vi "UHR-Fleezers Control (host) - Lorentz v2.vi"() -> ()   [LabVIEW 2014] (continued)
          tunnel: "Inject Pump 2" -> [_ w2660]
          frame False {
          }
          frame True {
            n1765 = local read "Flow rate (uL/h)"() -> (w2654:dbl)
            n1766 = Number To Decimal String(number=w2654) -> (decimal integer string=w2656:string)  [unwired: 1 in]
            n1767 = Concatenate Strings("on, flow rate", w2656) -> (w2655:string)
            n1768 = Select(t=w2655, s=w2660, f="off") -> (s? t:f=w2664:string)
            n1769 = local read "Time (s)"() -> (w2658:dbl)
            n1770 = local read "log file ref"() -> (w2659:refnum<file>)
            n1771 = Concatenate Strings("pump 2 ", w2664) -> (w2662:string)
            n1772 = call "write to event log.vi"("log file ref"=w2659, "time"=w2658, "input string"=w2662) -> ()  [unwired: 8 in]
          }
        }
      }
      event "Sample Channel\nFlow": Value Change {
        n1773 = event-data() -> ()  [unwired: 7 out]
        n1774 = disable-structure shown="Disabled" {
          disable-tunnel: w2682 -> [w2689 _]
          frame Disabled {
            n1775 = Select(t="irun" ("string"), s="Sample Channel\nFlow", f="stop" ("string")) -> (s? t:f=w2684:string)
            n1776 = Concatenate Strings(w2684, "\r") -> (w2687:string)
            n1777 = VISA Write(VISA resource name=w2689, write buffer=w2687) -> ()  [unwired: 1 in, 3 out]
          }
          frame Enabled {
          }
        }
      }
      event "Start Flow": Value Change {
        n1778 = event-data() -> ()  [unwired: 7 out]
        n1779 = disable-structure shown="Disabled" {
          disable-tunnel: w2690 -> [w2691 _]
          frame Disabled {
            n1780 = local write "Sample Channel\nFlow"(TRUE ("Sample Channel\nFlow")) -> ()
            n1781 = local write "Start Flow"(FALSE ("Start Flow")) -> ()
            n1782 = Concatenate Strings("irun" ("string"), "\r") -> (w2695:string)
            n1783 = VISA Write(VISA resource name=w2691, write buffer=w2695) -> ()  [unwired: 1 in, 3 out]
          }
          frame Enabled {
          }
        }
      }
      event "Stop Flow": Value Change {
        n1784 = event-data() -> ()  [unwired: 7 out]
        n1785 = disable-structure shown="Disabled" {
          disable-tunnel: w2697 -> [w2699 _]
          frame Disabled {
            w2698 = FALSE ("Stop Flow")
            n1786 = local write "Stop Flow"(w2698) -> ()
            n1787 = local write "Sample Channel\nFlow"(w2698) -> ()
            n1788 = Concatenate Strings("stop" ("string"), "\r") -> (w2701:string)
            n1789 = VISA Write(VISA resource name=w2699, write buffer=w2701) -> ()  [unwired: 1 in, 3 out]
          }
          frame Enabled {
          }
        }
      }
      event "Flow rate (uL/h)": Value Change {
        n1790 = event-data() -> ()  [unwired: 7 out]
        n1791 = disable-structure shown="Disabled" {
          disable-tunnel: w2703 -> [w2705 _]
          frame Disabled {
            n1792 = Number To Decimal String(number="Flow rate (uL/h)") -> (decimal integer string=w2709:string)  [unwired: 1 in]
            n1793 = Concatenate Strings("irate  " ("string"), w2709, " u/h" ("string"), "\r") -> (w2708:string)
            n1794 = VISA Write(VISA resource name=w2705, write buffer=w2708) -> ()  [unwired: 1 in, 3 out]
          }
          frame Enabled {
          }
        }
      }
      event "Flush Sample": Value Change {
        n1795 = event-data() -> ()  [unwired: 7 out]
        n1796 = disable-structure shown="Disabled" {
          disable-tunnel: ["Flush Sample" _] -> w2712
          disable-tunnel: w2711 -> [w2718 _]
          frame Disabled {
            n1797 = flat-sequence {
              tunnel: w2718 -> [w2759]
              tunnel: [w2739] -> w2722
              tunnel: [w2735] -> w2721
              tunnel: ["Volume (uL)"] -> w2717
              tunnel: ["Flush rate (uL/m)"] -> w2716
              tunnel: w2722 -> [w2763]
              tunnel: [w2763] -> w2720
              tunnel: w2721 -> [w2762]
              tunnel: w2720 -> [w2768]
              frame #0 {
                # "set paramaters (rate, volume) for flush, clear volume"
                n1798 = Number To Decimal String(number="Flush rate (uL/m)") -> (decimal integer string=w2755:string)  [unwired: 1 in]
                n1799 = Concatenate Strings("irate  " ("string"), w2755, " u/m" ("string"), "\r") -> (w2757:string)
                n1800 = VISA Write(VISA resource name=w2759, write buffer=w2757) -> (VISA resource name out=w2753:refnum<visa-resource-name>)  [unwired: 1 in, 2 out]
                n1801 = Reciprocal(x="Flush rate (uL/m)") -> (1/x=w2738:dbl)
                n1802 = Number To Decimal String(number="Volume (uL)") -> (decimal integer string=w2744:string)  [unwired: 1 in]
                n1803 = Multiply(x="Volume (uL)", y=w2738) -> (x*y=w2737:dbl)
                n1804 = Concatenate Strings("tvolume  " ("string"), w2744, " u" ("string"), "\r") -> (w2742:string)
                n1805 = Multiply(x=w2737, y=60000.0) -> (x*y=w2735:dbl)
                n1806 = VISA Write(VISA resource name=w2753, write buffer=w2742) -> (VISA resource name out=w2741:refnum<visa-resource-name>)  [unwired: 1 in, 2 out]
                n1807 = Concatenate Strings("cvolume" ("string"), "\r") -> (w2740:string)
                n1808 = VISA Write(VISA resource name=w2741, write buffer=w2740) -> (VISA resource name out=w2751:refnum<visa-resource-name>)  [unwired: 1 in, 2 out]
                n1809 = Concatenate Strings("irun" ("string"), "\r") -> (w2749:string)
                n1810 = VISA Write(VISA resource name=w2751, write buffer=w2749) -> (VISA resource name out=w2739:refnum<visa-resource-name>)  [unwired: 1 in, 2 out]
              }
              frame #1 {
                # "Have to wait until\nflow is done to reset\nrate"
                n1811 = Add(x=w2762, y=100.0) -> (x+y=w2761:dbl)
                n1812 = Wait (ms)(milliseconds to wait=w2761) -> ()  [unwired: 1 out]
              }
              frame #2 {
                # "reset flow rate to usual flow rate"
                n1813 = local read "Flow rate (uL/h)"() -> (w2774:dbl)
                n1814 = Number To Decimal String(number=w2774) -> (decimal integer string=w2772:string)  [unwired: 1 in]
                n1815 = Concatenate Strings("irate  " ("string"), w2772, " u/h" ("string"), "\r") -> (w2770:string)
                n1816 = VISA Write(VISA resource name=w2768, write buffer=w2770) -> (VISA resource name out=w2764:refnum<visa-resource-name>)  [unwired: 1 in, 2 out]
                n1817 = Concatenate Strings("cvolume" ("string"), "\r") -> (w2765:string)
                n1818 = VISA Write(VISA resource name=w2764, write buffer=w2765) -> ()  [unwired: 1 in, 3 out]
              }
            }
            n1819 = local read "Save Event Log?"() -> (w2714:bool)
            n1820 = local read "Saving..."() -> (w2713:bool)
            n1821 = And(x=w2714, y=w2713) -> (x .and. y?=w2715:bool)
            n1822 = case shown="True" w2715 {
              tunnel: w2717 -> [_ w2724]
              tunnel: w2716 -> [_ w2723]
              frame False {
              }
              frame True {
                n1823 = Number To Decimal String(number=w2724) -> (decimal integer string=w2728:string)  [unwired: 1 in]
                n1824 = Number To Decimal String(number=w2723) -> (decimal integer string=w2730:string)  [unwired: 1 in]
                n1825 = local read "log file ref"() -> (w2725:refnum<file>)
                n1826 = local read "Time (s)"() -> (w2726:dbl)
                n1827 = Concatenate Strings("pump 2 flushing ", w2728, " uL at ", w2730, " ul/min") -> (w2732:string)
                n1828 = call "write to event log.vi"("log file ref"=w2725, "time"=w2726, "input string"=w2732) -> ()  [unwired: 8 in]
              }
            }
          }
          frame Enabled {
          }
        }
      }
      event "Flush Pump 3": Value Change {
        n1829 = event-data() -> ()  [unwired: 7 out]
        n1830 = disable-structure shown="Disabled" {
          disable-tunnel: ["Flush Pump 3" _] -> w2776
          disable-tunnel: w2775 -> [w2782 _]
          frame Disabled {
            n1831 = flat-sequence {
              tunnel: w2782 -> [w2797]
              tunnel: ["Flush rate (uL/m) P3"] -> w2778
              tunnel: ["Volume (uL) P3"] -> w2777
              frame #0 {
                # "set paramaters (rate, volume) for flush, clear volume"
                n1832 = Number To Decimal String(number="Flush rate (uL/m) P3") -> (decimal integer string=w2817:string)  [unwired: 1 in]
                n1833 = local write "Inject Pump 3"(TRUE ("Inject Pump 3")) -> ()
                n1834 = Concatenate Strings("irate  " ("string"), w2817, " u/m" ("string"), "\r") -> (w2819:string)
                n1835 = VISA Write(VISA resource name=w2797, write buffer=w2819) -> (VISA resource name out=w2815:refnum<visa-resource-name>)  [unwired: 1 in, 2 out]
                n1836 = Reciprocal(x="Flush rate (uL/m) P3") -> (1/x=w2801:dbl)
                n1837 = Number To Decimal String(number="Volume (uL) P3") -> (decimal integer string=w2806:string)  [unwired: 1 in]
                n1838 = Multiply(x="Volume (uL) P3", y=w2801) -> (x*y=w2800:dbl)
                n1839 = Concatenate Strings("tvolume  " ("string"), w2806, " u" ("string"), "\r") -> (w2804:string)
                n1840 = Multiply(x=w2800, y=60.0) -> (x*y=→"HP3 Flush Time (s)":dbl)
                n1841 = VISA Write(VISA resource name=w2815, write buffer=w2804) -> (VISA resource name out=w2803:refnum<visa-resource-name>)  [unwired: 1 in, 2 out]
                n1842 = Concatenate Strings("cvolume" ("string"), "\r") -> (w2802:string)
                n1843 = VISA Write(VISA resource name=w2803, write buffer=w2802) -> (VISA resource name out=w2813:refnum<visa-resource-name>)  [unwired: 1 in, 2 out]
                n1844 = Concatenate Strings("irun" ("string"), "\r") -> (w2811:string)
                n1845 = VISA Write(VISA resource name=w2813, write buffer=w2811) -> ()  [unwired: 1 in, 3 out]
              }
              frame #1 {
                "Flushing P3" <- TRUE ("Flushing P3")
              }
            }
            n1846 = local read "Save Event Log?"() -> (w2780:bool)
            n1847 = local read "Saving..."() -> (w2781:bool)
            n1848 = And(x=w2780, y=w2781) -> (x .and. y?=w2779:bool)
            n1849 = case shown="True" w2779 {
              tunnel: w2778 -> [_ w2785]
              tunnel: w2777 -> [_ w2784]
              frame False {
              }
              frame True {
                n1850 = Number To Decimal String(number=w2784) -> (decimal integer string=w2789:string)  [unwired: 1 in]
                n1851 = Number To Decimal String(number=w2785) -> (decimal integer string=w2791:string)  [unwired: 1 in]
                n1852 = local read "log file ref"() -> (w2786:refnum<file>)
                n1853 = local read "Time (s)"() -> (w2787:dbl)
                n1854 = Concatenate Strings("pump 3 flushing ", w2789, " uL at ", w2791, " ul/min") -> (w2793:string)
                n1855 = call "write to event log.vi"("log file ref"=w2786, "time"=w2787, "input string"=w2793) -> ()  [unwired: 8 in]
              }
            }
          }
          frame Enabled {
          }
        }
      }
      event "Flush Pump 1": Value Change {
        n1856 = event-data() -> ()  [unwired: 7 out]
        n1857 = disable-structure shown="Disabled" {
          disable-tunnel: ["Flush Pump 1" _] -> w2823
          disable-tunnel: w2822 -> [w2829 _]
          frame Disabled {
            n1858 = flat-sequence {
              tunnel: [w2850] -> w2831
              tunnel: w2829 -> [w2845]
              tunnel: ["Volume (uL) P1"] -> w2825
              tunnel: ["Flush rate (uL/m) P1"] -> w2824
              tunnel: w2831 -> [_]
              frame #0 {
                # "set paramaters (rate, volume) for flush, clear volume"
                n1859 = local write "Inject Pump 1"(TRUE ("Inject Pump 1")) -> ()
                n1860 = Number To Decimal String(number="Flush rate (uL/m) P1") -> (decimal integer string=w2866:string)  [unwired: 1 in]
                n1861 = Concatenate Strings("irate  " ("string"), w2866, " u/m" ("string"), "\r") -> (w2868:string)
                n1862 = VISA Write(VISA resource name=w2845, write buffer=w2868) -> (VISA resource name out=w2864:refnum<visa-resource-name>)  [unwired: 1 in, 2 out]
                n1863 = Reciprocal(x="Flush rate (uL/m) P1") -> (1/x=w2849:dbl)
                n1864 = Number To Decimal String(number="Volume (uL) P1") -> (decimal integer string=w2855:string)  [unwired: 1 in]
                n1865 = Multiply(x="Volume (uL) P1", y=w2849) -> (x*y=w2848:dbl)
                n1866 = Concatenate Strings("tvolume  " ("string"), w2855, " u" ("string"), "\r") -> (w2853:string)
                n1867 = Multiply(x=w2848, y=60.0) -> (x*y=→"HP1 Flush Time (s)":dbl)
                n1868 = VISA Write(VISA resource name=w2864, write buffer=w2853) -> (VISA resource name out=w2852:refnum<visa-resource-name>)  [unwired: 1 in, 2 out]
                n1869 = Concatenate Strings("cvolume" ("string"), "\r") -> (w2851:string)
                n1870 = VISA Write(VISA resource name=w2852, write buffer=w2851) -> (VISA resource name out=w2862:refnum<visa-resource-name>)  [unwired: 1 in, 2 out]
                n1871 = Concatenate Strings("irun" ("string"), "\r") -> (w2860:string)
                n1872 = VISA Write(VISA resource name=w2862, write buffer=w2860) -> (VISA resource name out=w2850:refnum<visa-resource-name>)  [unwired: 1 in, 2 out]
              }
              frame #1 {
                "Flushing P1" <- TRUE ("Flushing P3")
              }
            }
            n1873 = local read "Saving..."() -> (w2826:bool)
            n1874 = local read "Save Event Log?"() -> (w2827:bool)
            n1875 = And(x=w2827, y=w2826) -> (x .and. y?=w2828:bool)
            n1876 = case shown="True" w2828 {
              tunnel: w2825 -> [_ w2834]
              tunnel: w2824 -> [_ w2833]
              frame False {
              }
              frame True {
                n1877 = Number To Decimal String(number=w2834) -> (decimal integer string=w2838:string)  [unwired: 1 in]
                n1878 = Number To Decimal String(number=w2833) -> (decimal integer string=w2836:string)  [unwired: 1 in]
                n1879 = local read "log file ref"() -> (w2840:refnum<file>)
                n1880 = local read "Time (s)"() -> (w2841:dbl)
                n1881 = Concatenate Strings("pump 1 flushing ", w2838, " uL at ", w2836, " ul/min") -> (w2832:string)
                n1882 = call "write to event log.vi"("log file ref"=w2840, "time"=w2841, "input string"=w2832) -> ()  [unwired: 8 in]
              }
            }
          }
          frame Enabled {
          }
        }
      }
      event "Clear Volume": Value Change {
        n1883 = event-data() -> ()  [unwired: 7 out]
        n1884 = disable-structure shown="Disabled" {
          disable-tunnel: ["Clear Volume" _] -> w2872
          disable-tunnel: w2871 -> [w2873 _]
          frame Disabled {
            n1885 = Concatenate Strings("cvolume" ("string"), "\r") -> (w2874:string)
            n1886 = VISA Write(VISA resource name=w2873, write buffer=w2874) -> ()  [unwired: 1 in, 3 out]
          }
          frame Enabled {
          }
        }
      }
      event "Clear Volume P3": Value Change {
        n1887 = event-data() -> ()  [unwired: 7 out]
        n1888 = disable-structure shown="Disabled" {
          disable-tunnel: w2878 -> [w2880 _]
          frame Disabled {
            n1889 = Concatenate Strings("cvolume" ("string"), "\r") -> (w2881:string)
            n1890 = VISA Write(VISA resource name=w2880, write buffer=w2881) -> ()  [unwired: 1 in, 3 out]
            n1891 = local write "Clear Volume P3"(FALSE ("Clear Volume P3")) -> ()
          }
          frame Enabled {
          }
        }
      }
      event "Clear Volume P1": Value Change {
        n1892 = event-data() -> ()  [unwired: 7 out]
        n1893 = disable-structure shown="Disabled" {
          disable-tunnel: w2884 -> [w2886 _]
          frame Disabled {
            n1894 = Concatenate Strings("cvolume" ("string"), "\r") -> (w2887:string)
            n1895 = local write "Clear Volume P1"(FALSE ("Clear Volume P1")) -> ()
            n1896 = VISA Write(VISA resource name=w2886, write buffer=w2887) -> ()  [unwired: 1 in, 3 out]
          }
          frame Enabled {
          }
        }
      }
      event "Display On P3": Value Change {
        n1897 = event-data() -> ()  [unwired: 7 out]
        n1898 = disable-structure shown="Disabled" {
          disable-tunnel: w2890 -> [w2891 _]
          frame Disabled {
            n1899 = Select(t="dim 100", s="Display On P3", f="dim 0") -> (s? t:f=w2894:string)
            n1900 = Concatenate Strings(w2894, "\r") -> (w2896:string)
            n1901 = VISA Write(VISA resource name=w2891, write buffer=w2896) -> ()  [unwired: 1 in, 3 out]
          }
          frame Enabled {
          }
        }
      }
      event "Display On P1": Value Change {
        n1902 = event-data() -> ()  [unwired: 7 out]
        n1903 = disable-structure shown="Disabled" {
          disable-tunnel: w2898 -> [w2899 _]
          frame Disabled {
            n1904 = Select(t="dim 100", s="Display On P1", f="dim 0") -> (s? t:f=w2902:string)
            n1905 = Concatenate Strings(w2902, "\r") -> (w2904:string)
            n1906 = VISA Write(VISA resource name=w2899, write buffer=w2904) -> ()  [unwired: 1 in, 3 out]
          }
          frame Enabled {
          }
        }
      }
      event "Retract Pump 3": Value Change {
        n1907 = event-data() -> ()  [unwired: 7 out]
        n1908 = disable-structure shown="Disabled" {
          disable-tunnel: w2906 -> [w2907 _]
          frame Disabled {
            n1909 = local write "Retract Pump 3"(FALSE ("Retract Pump 3")) -> ()
            n1910 = case shown="True" "Retract Pump 3" {
              tunnel: w2907 -> [_ w2910]
              frame False {
              }
              frame True {
                n1911 = Number To Decimal String(number="Retract Rate (uL/m)") -> (decimal integer string=w2928:string)  [unwired: 1 in]
                n1912 = Concatenate Strings("wrate  " ("string"), w2928, " u/m" ("string"), "\r") -> (w2930:string)
                n1913 = VISA Write(VISA resource name=w2910, write buffer=w2930) -> (VISA resource name out=w2921:refnum<visa-resource-name>)  [unwired: 1 in, 2 out]
                n1914 = Number To Decimal String(number="Retract Vol 3 (uL)") -> (decimal integer string=w2923:string)  [unwired: 1 in]
                n1915 = Concatenate Strings("tvolume  " ("string"), w2923, " u" ("string"), "\r") -> (w2920:string)
                n1916 = VISA Write(VISA resource name=w2921, write buffer=w2920) -> (VISA resource name out=w2916:refnum<visa-resource-name>)  [unwired: 1 in, 2 out]
                n1917 = Concatenate Strings("cvolume" ("string"), "\r") -> (w2917:string)
                n1918 = VISA Write(VISA resource name=w2916, write buffer=w2917) -> (VISA resource name out=w2911:refnum<visa-resource-name>)  [unwired: 1 in, 2 out]
                n1919 = Concatenate Strings("wrun" ("string"), "\r") -> (w2912:string)
                n1920 = VISA Write(VISA resource name=w2911, write buffer=w2912) -> ()  [unwired: 1 in, 3 out]
              }
            }
          }
          frame Enabled {
          }
        }
      }
      event "Retract Pump 1": Value Change {
        n1921 = event-data() -> ()  [unwired: 7 out]
        n1922 = disable-structure shown="Disabled" {
          disable-tunnel: w2932 -> [w2933 _]
          frame Disabled {
            n1923 = local write "Retract Pump 1"(FALSE ("Retract Pump 1")) -> ()
            n1924 = case shown="True" "Retract Pump 1" {
              tunnel: w2933 -> [_ w2938]
              frame False {
              }
              frame True {
                n1925 = local read "Retract Rate (uL/m)"() -> (w2936:dbl)
                n1926 = Number To Decimal String(number=w2936) -> (decimal integer string=w2954:string)  [unwired: 1 in]
                n1927 = Concatenate Strings("wrate  " ("string"), w2954, " u/m" ("string"), "\r") -> (w2956:string)
                n1928 = VISA Write(VISA resource name=w2938, write buffer=w2956) -> (VISA resource name out=w2948:refnum<visa-resource-name>)  [unwired: 1 in, 2 out]
                n1929 = Number To Decimal String(number="Retract Vol 1 (uL)") -> (decimal integer string=w2950:string)  [unwired: 1 in]
                n1930 = Concatenate Strings("tvolume  " ("string"), w2950, " u" ("string"), "\r") -> (w2947:string)
                n1931 = VISA Write(VISA resource name=w2948, write buffer=w2947) -> (VISA resource name out=w2944:refnum<visa-resource-name>)  [unwired: 1 in, 2 out]
                n1932 = Concatenate Strings("cvolume" ("string"), "\r") -> (w2945:string)
                n1933 = VISA Write(VISA resource name=w2944, write buffer=w2945) -> (VISA resource name out=w2939:refnum<visa-resource-name>)  [unwired: 1 in, 2 out]
                n1934 = Concatenate Strings("wrun" ("string"), "\r") -> (w2940:string)
                n1935 = VISA Write(VISA resource name=w2939, write buffer=w2940) -> ()  [unwired: 1 in, 3 out]
              }
            }
          }
          frame Enabled {
          }
        }
      }
      event "Flip Green Filter": Value Change {
        n1936 = event-data() -> ()  [unwired: 7 out]
        n1937 = Not(x="Flip Green Filter") -> (.not. x?=w2959:bool)
        n1938 = local write "Flip Green Filter"(w2959) -> ()
        n1939 = flat-sequence {
          tunnel: [w2968] -> w2964
          tunnel: [w2967] -> w2963
          tunnel: w2958 -> [w2966]
          tunnel: [w2971] -> w2962
          tunnel: w2964 -> [w2971]
          tunnel: [w2970] -> w2961
          tunnel: w2963 -> [w2970]
          tunnel: w2962 -> [w2975]
          tunnel: w2961 -> [w2974]
          tunnel: [w2973] -> w2965
          frame #0 {
            n1940 = xnode "Read/Write Control"("FPGA VI Reference In"=w2966, "Green Filter Flipper"=TRUE) -> ("FPGA VI Reference Out"=w2968:T31, "error out"=w2967:errorcluster)  [unwired: 1 in]
          }
          frame #1 {
            n1941 = Wait (ms)(milliseconds to wait=u32 100) -> ()  [unwired: 1 out]
          }
          frame #2 {
            n1942 = xnode "Read/Write Control"("FPGA VI Reference In"=w2975, "error in"=w2974, "Green Filter Flipper"=FALSE) -> ("error out"=w2973:errorcluster)  [unwired: 1 out]
          }
        }
      }
      event "Pump 1 contents", "Pump 3 contents": Value Change {
        n1943 = event-data() -> ()  [unwired: 7 out]
        n1944 = local read "Pump 1 contents"() -> (→"Pump 1 cont disp":string)
        n1945 = local read "Pump 3 contents"() -> (→"Pump 3 cont disp":string)
      }
      event "Reset Trap Pos. FB": Value Change {
        n1946 = event-data() -> ()  [unwired: 7 out]
        n1947 = xnode "Read/Write Control"("FPGA VI Reference In"=w2979, "Trap Pos. FB Reset"="Reset Trap Pos. FB") -> ()  [unwired: 1 in, 2 out]
      }
      event "Rem fb disp offset": Value Change {
        n1948 = event-data() -> ()  [unwired: 7 out]
        n1949 = local write "Rem fb disp offset"(FALSE ("Rem fb disp offset")) -> ()
        n1950 = local read "Mean T1 Position (nm)"() -> (w2982:dbl)
        n1951 = local read "FB Trap Pos Offset"() -> (w2983:dbl)
        n1952 = Subtract(x=w2983, y=w2982) -> (x-y=w2981:dbl)
        n1953 = local write "FB Trap Pos Offset"(w2981) -> ()
      }
      event "Threshold (nm)": Value Change {
        n1954 = event-data() -> ()  [unwired: 7 out]
        n1955 = flat-sequence {
          tunnel: [w2988] -> w2986
          tunnel: w2985 -> [w2987]
          tunnel: w2986 -> [w2999]
          frame #0 {
            n1956 = xnode "Read/Write Control"("FPGA VI Reference In"=w2987) -> ("FPGA VI Reference Out"=w2991:T31, "error out"=w2990:errorcluster, "FPGA TTrig Thresh"=w2992:i64)  [unwired: 1 in]
            n1957 = local read "Threshold stored (nm)"() -> (w2998:dbl)
            n1958 = local read "Threshold (nm)"() -> (w2988:dbl)
            n1959 = local read "AOM X Cal (nm/MHz)"() -> (w2996:dbl)
            n1960 = Subtract(x=w2988, y=w2998) -> (x-y=w2997:dbl)
            n1961 = Divide(x=w2997, y=w2996) -> (x/y=w2994:dbl)
            n1962 = call "IR AOM freq to word.vi"("Frequency In (MHz)"=w2994) -> ("Frequency Word Out (double)"=w2995:dbl)
            n1963 = To Quad Integer(1:w2995) -> (0:w2993:i64)
            n1964 = Add(x=w2992, y=w2993) -> (x+y=w2989:i64)
            n1965 = xnode "Read/Write Control"("FPGA VI Reference In"=w2991, "error in"=w2990, "FPGA TTrig Thresh"=w2989) -> ()  [unwired: 2 out]
          }
          frame #1 {
            "Threshold stored (nm)" <- w2999
          }
        }
      }
      event "FB Trig Integrate": Value Change {
        n1966 = event-data() -> ()  [unwired: 7 out]
        n1967 = local read "FB Trig Integrate"() -> (w3002:u32)
        n1968 = xnode "Read/Write Control"("FPGA VI Reference In"=w3000, "FB Trig Integrate"=w3002) -> ("error out"=w3001:errorcluster)  [unwired: 1 in, 1 out]
      }
      event "11": Value Change {
        n1969 = event-data() -> ()  [unwired: 7 out]
        n1970 = local read "11"() -> (w3003:bool)
        n1971 = case shown="True" w3003 {
          frame False {
          }
          frame True {
            n1972 = local read "Messages"() -> (w3005:string)
            n1973 = call "Update messages.vi"("Message to add"="You kicked it up to 11!", "Old message string"=w3005) -> ("New message string"=w3006:string)
            n1974 = call <vilib>:"Beep.vi"() -> ()  [unwired: 12 in]
            n1975 = local write "Messages"(w3006) -> ()
          }
        }
      }
      event "Trap Pos. FB ON": Value Change {
        w3013 = 6.0  # clock mult.
        w3012 = 49152000.0  # TCXO frequ.
        n1976 = event-data() -> ()  [unwired: 7 out]
        n1977 = xnode "Read/Write Control"("FPGA VI Reference In"=w3007) -> ("FPGA VI Reference Out"=w3009:T31, "BD1 Frequency Out 1"=w3010:u64)  [unwired: 1 in, 1 out]
        n1978 = To Double Precision Float(number=w3010) -> (double precision float=w3014:dbl)
        n1979 = Multiply(x=w3012, y=w3013) -> (x*y=w3015:dbl)
        n1980 = Multiply(x=w3014, y=w3015) -> (x*y=w3016:dbl)
        n1981 = Scale By Power Of 2(n=-48, x=w3016) -> (x*2^n=w3018:dbl)
        n1982 = Divide(x=w3018, y=1000000.0) -> (x/y=w3011:dbl)
        n1983 = flat-sequence {
          tunnel: w3009 -> [w3024]
          tunnel: [w3023] -> w3020
          tunnel: "Trap Pos. FB ON" -> [w3022]
          tunnel: w3010 -> [w3021]
          tunnel: w3020 -> [w3030]
          tunnel: "Trap Pos. FB ON" -> [w3029]
          tunnel: w3011 -> [w3032]
          tunnel: "Trap Pos. FB ON" -> [w3031]
          frame #0 {
            n1984 = case shown="False" w3022 {
              tunnel: w3024 -> [w3026 w3028]
              tunnel: [w3027 w3028] -> w3023
              tunnel: w3021 -> [w3025 _]
              frame False {
                n1985 = xnode "Read/Write Control"("FPGA VI Reference In"=w3026, "BD 1 Frequency 1"=w3025) -> ("FPGA VI Reference Out"=w3027:T31)  [unwired: 1 in, 1 out]
              }
              frame True {
              }
            }
          }
          frame #1 {
            n1986 = xnode "Read/Write Control"("FPGA VI Reference In"=w3030, "Force feedback"=w3029) -> ()  [unwired: 1 in, 2 out]
          }
          frame #2 {
            n1987 = case shown="False" w3031 {
              tunnel: w3032 -> [w3033 _]
              frame False {
                n1988 = property on="BD 1 Frequency 1 (MHz)" class="DigNum (strict)"("Val(Sgnl)"=w3033) -> ()  [unwired: 2 in, 2 out]
              }
              frame True {
              }
            }
          }
        }
      }
      event "Remove Action Offset": Value Change {
        n1989 = event-data() -> ()  [unwired: 7 out]
        n1990 = local write "Remove Action Offset"(FALSE ("Remove Action Offset")) -> ()
        n1991 = local read "Trap Pos. FB Mult Factor"() -> (w3039:i64)
        n1992 = local read "Trap Pos FB Action"() -> (w3037:i64)
        n1993 = local read "Trap Pos. FB Offset Factor"() -> (w3035:i64)
        n1994 = Multiply(x=w3039, y=w3037) -> (x*y=w3038:i64)
        n1995 = Add(x=w3038, y=w3035) -> (x+y=w3036:i64)
        n1996 = local write "Trap Pos. FB Offset Factor"(w3036) -> ()
        n1997 = xnode "Read/Write Control"("FPGA VI Reference In"=w3034, "Trap Pos. FB Offset Factor"=w3036) -> ()  [unwired: 1 in, 2 out]
      }
      event "Remove Unwinding Offset": Value Change {
        n1998 = event-data() -> ()  [unwired: 7 out]
        n1999 = local write "Remove Unwinding Offset"(FALSE ("Remove Action Offset")) -> ()
        n2000 = local read "Trap Pos. FB Mult Factor"() -> (w3053:i64)
        n2001 = local read "Trap Pos FB Action"() -> (w3051:i64)
        n2002 = local read "Trap Pos. FB Offset Factor"() -> (w3050:i64)
        n2003 = Multiply(x=w3053, y=w3051) -> (x*y=w3052:i64)
        n2004 = local read "Trap Pos. FB Mult Factor"() -> (w3049:i64)
        n2005 = Add(x=w3052, y=w3050) -> (x+y=w3043:i64)
        n2006 = Multiply(x=32768, y="factor") -> (x*y=w3046:dbl)
        n2007 = Multiply(x=w3046, y=w3049) -> (x*y=w3048:dbl)
        n2008 = Subtract(x=w3043, y=w3048) -> (x-y=w3047:dbl)
        n2009 = To Quad Integer(1:w3047) -> (0:w3042:i64)
        n2010 = xnode "Read/Write Control"("FPGA VI Reference In"=w3041, "Trap Pos. FB Offset Factor"=w3042) -> ()  [unwired: 1 in, 2 out]
        n2011 = local write "Trap Pos. FB Offset Factor"(w3042) -> ()
      }
      event "Trap Pos. FB Range", "Trap Pos. FB Gains", "Trap Pos. FB Mult Factor", "Trap Pos. FB Offset Factor", "Trap Pos FB Negate Action", "Trap Pos FB Monitor\nT1 or T2", "Differential FB?", "Negate Diff?": Value Change {
        n2012 = event-data() -> ()  [unwired: 7 out]
        n2013 = local read "Negate Diff?"() -> (w3058:bool)
        n2014 = xnode "Read/Write Control"("FPGA VI Reference In"=w3057, "Trap Pos. FB Gains"="Trap Pos. FB Gains", "Trap pos. FB Range"="Trap Pos. FB Range", "Trap Pos. FB Mult Factor"="Trap Pos. FB Mult Factor", "Trap Pos. FB Offset Factor"="Trap Pos. FB Offset Factor", "Trap Pos FB Negate Action"="Trap Pos FB Negate Action", "Trap Pos FB Monitor T1 or T2"="Trap Pos FB Monitor\nT1 or T2", "AI1 X Scale"="Trap Pos. AI1 X Pre-scale", "Negate Diff?"=w3058, "Diff FB Measurement?"="Differential FB?") -> ()  [unwired: 1 in, 2 out]
      }
      event "Trap Pos FB SP", "Trap Pos FB SP 2", "Use SP 2": Value Change {
        n2015 = event-data() -> ()  [unwired: 7 out]
        n2016 = Select(t="Trap Pos FB SP 2", s="Use SP 2", f="Trap Pos FB SP") -> (s? t:f=w3066:fxp<+/-,16,1>)
        n2017 = xnode "Read/Write Control"("FPGA VI Reference In"=w3065, "Trap Pos. FB SP"=w3066) -> ()  [unwired: 1 in, 2 out]
      }
      event "Offset SP2 from SP1": Value Change {
        n2018 = event-data() -> ()  [unwired: 7 out]
        n2019 = local read "Trap Pos FB SP"() -> (w3072:fxp<+/-,16,1>)
        n2020 = Add(x=w3072, y="SP2 Offset") -> (x+y=w3070:fxp<+/-,16,1>)
        n2021 = property on="Trap Pos FB SP 2" class="DigNum (strict)"("Val(Sgnl)"=w3070) -> ()  [unwired: 2 in, 2 out]
        n2022 = local write "Offset SP2 from SP1"(FALSE ("Offset SP2 from SP1")) -> ()
      }
      event "Set Reading to\nSetpoint": Value Change {
        # "This is the actual PID input signal"
        n2023 = event-data() -> ()  [unwired: 7 out]
        n2024 = local write "Set Reading to\nSetpoint"(FALSE ("Set SP to Reading")) -> ()
        n2025 = xnode "Read/Write Control"("FPGA VI Reference In"=w3076) -> ("FPGA VI Reference Out"=w3079:T31, "error out"=w3078:errorcluster, "Trap Pos FB Int-Norm Signal"=w3077:fxp<+/-,16,1>, "BD1 Frequency Out 1"=w3075:u64)  [unwired: 1 in]
        n2026 = local read "Differential FB?"() -> (w3080:bool)
        n2027 = case shown="False" w3080 {
          tunnel: [w3109 w3116] -> w3074
          tunnel: w3077 -> [w3107 w3116]
          frame False {
            n2028 = local read "Trap Pos FB Monitor\nT1 or T2"() -> (w3112:bool)
            n2029 = local read "Trap X AI1 (DMA)"() -> (w3115:T16)
            n2030 = Unbundle By Name(w3115) -> ("Set 1"=w3114:fxp<+/-,16,1>, "Set 2"=w3113:fxp<+/-,16,1>)
            n2031 = Select(t=w3114, s=w3112, f=w3113) -> (s? t:f=w3111:fxp<+/-,16,1>)
            n2032 = Not(x="Set SP Using...") -> (.not. x?=w3108:bool)
            n2033 = Select(t=w3107, s=w3108, f=w3111) -> (s? t:f=w3109:fxp<+/-,16,1>)
          }
          frame True {
          }
        }
        n2034 = disable-structure shown="Disabled" {
          disable-tunnel: _ -> [w3085 _]
          disable-tunnel: w3075 -> [w3084 _]
          disable-tunnel: w3074 -> [w3083 _]
          frame Disabled {
            n2035 = case shown="True" w3085 {
              tunnel: [w3086 w3088] -> w3082
              tunnel: w3083 -> [w3086 w3087]
              tunnel: w3084 -> [_ w3106]
              frame False {
              }
              frame True {
                w3104 = 6.0  # clock mult.
                w3105 = 49152000.0  # TCXO frequ.
                # "Added by Ronen - for the real time\nchange of the setpoint to accomodate \nchanges in the offset."
                n2036 = To Double Precision Float(number=w3106) -> (double precision float=w3103:dbl)
                n2037 = local read "BD 1 Frequency 2 (MHz)"() -> (w3096:dbl)
                n2038 = Multiply(x=w3105, y=w3104) -> (x*y=w3102:dbl)
                n2039 = Multiply(x=w3103, y=w3102) -> (x*y=w3101:dbl)
                n2040 = local read "Offset file step size"() -> (w3094:dbl)
                n2041 = Scale By Power Of 2(n=-48, x=w3101) -> (x*2^n=w3099:dbl)
                n2042 = Divide(x=w3099, y=1000000.0) -> (x/y=w3097:dbl)
                n2043 = Subtract(x=w3096, y=w3097) -> (x-y=w3095:dbl)
                n2044 = Divide(x=w3095, y=w3094) -> (x/y=w3093:dbl)
                n2045 = local read item#-1() -> (w3091)
                n2046 = To Long Integer(number=w3093) -> (32bit integer=w3092:i32)
                n2047 = Index Array(array=w3091, index=w3092) -> (element=w3090)
                n2048 = To Fixed-Point(number=w3090) -> (fixed-point=w3089:fxp<+/-,16,1>)  [unwired: 1 in]
                n2049 = Add(x=w3087, y=w3089) -> (x+y=w3088:fxp<+/-,17,2>)
              }
            }
            "Offset corrected setpoint" <- w3082
          }
          frame Enabled {
          }
        }
        n2050 = local write "Trap Pos FB SP"(w3074) -> ()
        n2051 = xnode "Read/Write Control"("FPGA VI Reference In"=w3079, "error in"=w3078, "Trap Pos. FB SP"=w3074) -> ()  [unwired: 2 out]
      }
      event "Trap Pos. FB Out Scale 2^n": Value Change {
        n2052 = event-data() -> ()  [unwired: 7 out]
        n2053 = Scale By Power Of 2(n="Trap Pos. FB Out Scale 2^n", x=ext 1.0) -> (x*2^n=w3117:ext)
        n2054 = property on="Trap Pos. FB Mult Factor" class="DigNum (strict)"("Val(Sgnl)"=w3117) -> ()  [unwired: 2 in, 2 out]
      }
      event "Trap Pos FB Int Count": Value Change {
        n2055 = event-data() -> ()  [unwired: 7 out]
        n2056 = xnode "Read/Write Control"("FPGA VI Reference In"=w3120, "Trap Pos FB Int Count"="Trap Pos FB Int Count") -> ()  [unwired: 1 in, 2 out]
      }
      event "Display Saved Data": Value Change {
        n2057 = event-data() -> ()  [unwired: 7 out]
        n2058 = case shown="\"Amp Current\"" "Display Saved Data" {
          frame "Bead Seperation", Default {
            n2059 = property on="Amp current" class="WFGraph (strict)"("Visible"=FALSE) -> ()  [unwired: 2 in, 2 out]
            n2060 = property on="Trap Delta Graph" class="WFGraph (strict)"("Visible"=TRUE) -> ()  [unwired: 2 in, 2 out]
            n2061 = property on="Saved trap pos" class="WFGraph (strict)"("Visible"=FALSE) -> ()  [unwired: 2 in, 2 out]
          }
          frame "Amp Current" {
            n2062 = property on="Saved trap pos" class="WFGraph (strict)"("Visible"=FALSE) -> ()  [unwired: 2 in, 2 out]
            n2063 = property on="Trap Delta Graph" class="WFGraph (strict)"("Visible"=FALSE) -> ()  [unwired: 2 in, 2 out]
            n2064 = property on="Amp current" class="WFGraph (strict)"("Visible"=TRUE) -> ()  [unwired: 2 in, 2 out]
          }
          frame "Trap Position" {
            n2065 = property on="Saved trap pos" class="WFGraph (strict)"("Visible"=TRUE) -> ()  [unwired: 2 in, 2 out]
            n2066 = property on="Trap Delta Graph" class="WFGraph (strict)"("Visible"=FALSE) -> ()  [unwired: 2 in, 2 out]
            n2067 = property on="Amp current" class="WFGraph (strict)"("Visible"=FALSE) -> ()  [unwired: 2 in, 2 out]
          }
        }
      }
      event "Calibration": Value Change {
        n2068 = event-data() -> ()  [unwired: 7 out]
        n2069 = local read "X or Y?"() -> (w3148:bool)
        n2070 = local read "Calibration"() -> (w3145:u16)
        n2071 = Select(t="X" ("Label.Text"), s=w3148, f="Y" ("Label.Text")) -> (s? t:f=w3142:string)
        n2072 = case shown="0, Default" w3145 {
          tunnel: ["Position (V)" ("Label.Text") "Position (nm)" ("Label.Text") "Force (pN)" ("Label.Text")] -> w3139
          tunnel: [" (V)" ("Label.Text") " (nm)" ("Label.Text") " (pN)" ("Label.Text")] -> w3136
          frame 0, Default {
          }
          frame 1 {
          }
          frame 2 {
          }
        }
        n2073 = Concatenate Strings("T1 " ("Label.Text"), w3142) -> (w3138:string)
        n2074 = Concatenate Strings("T2 " ("Label.Text"), w3142) -> (w3137:string)
        n2075 = property on="Force" class="WFChart (strict)"("YScale.NameLbl.Text"=w3139) -> ()  [unwired: 2 in, 2 out]
        n2076 = Concatenate Strings("Mean" ("Label.Text"), w3136) -> (w3135:string)
        n2077 = Concatenate Strings(w3138, w3136) -> (w3134:string)
        n2078 = Concatenate Strings(w3137, w3136) -> (w3133:string)
        n2079 = Concatenate Strings("Difference" ("Label.Text"), w3136) -> (w3132:string)
        n2080 = property on="Mean" class="DigNum (strict)"("Caption.Text"=w3135) -> ()  [unwired: 2 in, 2 out]
        n2081 = property on="T1 X" class="DigNum (strict)"("Caption.Text"=w3134) -> ()  [unwired: 2 in, 2 out]
        n2082 = property on="T2 X" class="DigNum (strict)"("Caption.Text"=w3133) -> ()  [unwired: 2 in, 2 out]
        n2083 = property on="Difference" class="DigNum (strict)"("Caption.Text"=w3132) -> ()  [unwired: 2 in, 2 out]
      }
      event "Base N trap periods", "Period scale factor", "Trap osc amp (MHz)", "Cal sets to save", "# Samples/trap", "Total Counts (ticks)": Value Change {
        w3155 = 1.0
        w3161 = u32 0 ("y")
        # "scales 0 to 2pi"
        # "Create vector of trap offset (oscillation) values."
        # "Compute oscillation period as a multiple of the trap period. Should also fit nicely as a factor of the DMA period.\nCompare ticks for accurate commensurability check."
        # "Oscillation frequency needs to be commensurate\nwith the data save time."
        # "Be commensurate with total save time/100 (or so). That way you are guaranteed you can average spectra at least 100x."
        n2084 = event-data() -> ()  [unwired: 7 out]
        n2085 = local read "Total Counts (ticks)"() -> (w3177:u16)
        n2086 = To Unsigned Long Integer(number=w3177) -> (unsigned 32bit integer=w3187:u32)
        n2087 = Multiply "Base osc period (ticks)"(x=w3187, y="Base N trap periods") -> (x*y=w3178:u32)
        n2088 = local read "# Samples/trap"() -> (w3182:u32)
        n2089 = Multiply "Scaled osc period (ticks)"(x=w3178, y="Period scale factor") -> (x*y=w3179:dbl)
        n2090 = Multiply(x="Base N trap periods", y="Period scale factor") -> ()  [unwired: 1 out]
        n2091 = local read "Cal sets to save"() -> (w3183:u32)
        n2092 = To Unsigned Quad Integer(1:w3179) -> (0:w3169:u64)
        n2093 = for "vector 0 to N -1" {
          N: w3155 -> [_]
          tunnel: [w3204] -> w3175 mode=indexing
          i -> [w3204]
        }
        n2094 = Multiply "Ticks/DMA"(x=w3182, y=w3187) -> (x*y=w3186:u32)
        n2095 = Multiply "Scaled osc period (s)"(x=w3169, y=2.5e-08) -> (x*y=w3181:dbl)
        "Trap OSC Period (s)" <- w3181
        n2096 = Reciprocal(x=w3181) -> (1/x=→"A cal freq (Hz)":dbl)
        n2097 = Multiply(x=w3175, y=6.283185307179586) -> (x*y=w3190:dbl[])
        n2098 = Quotient & Remainder(x=w3186, y=w3169) -> (x-y*floor(x/y)=w3162:u64, floor(x/y)=→"N osc / DMA":u64)
        "DMA remainder" <- w3162
        n2099 = Multiply "Total trap ticks"(x=w3183, y=w3186) -> (x*y=w3170:u32)
        n2100 = Divide(x=w3190, y=w3155) -> (x/y=w3191:dbl[])
        n2101 = Sine(x=w3191) -> (sin(x)=w3192:dbl[])
        n2102 = Quotient & Remainder(x=w3170, y=100) -> (x-y*floor(x/y)=w3165:u32, floor(x/y)=w3185:u32)
        "Total save/100 remainder" <- w3165
        n2103 = Multiply "Single period osc vector"(x=w3192, y="Trap osc amp (MHz)") -> (x*y=w3168:dbl[])
        n2104 = Quotient & Remainder(x=w3185, y=w3169) -> (x-y*floor(x/y)=w3164:u64, floor(x/y)=→"N osc/ (total save/100)":u64)
        "(total save/100) /osc period remainder" <- w3164
        n2105 = Quotient & Remainder(x=w3170, y=w3169) -> (x-y*floor(x/y)=w3163:u64)  [unwired: 1 out]
        "N trap osc periods per save remainder" <- w3163
        n2106 = call "IR AOM freq to word - vec.vi"("Frequency In (double vec, MHz)"=w3168) -> ("Frequency Word Out"=w3167:dbl[])
        n2107 = To Quad Integer(1:w3167) -> (0:w3166:i64[])
        n2108 = disable-structure shown="Disabled" {
          disable-tunnel: w3174 -> [w3196 _]
          disable-tunnel: w3166 -> [w3194 _]
          frame Disabled {
            n2109 = xnode "Read/Write Control"("FPGA VI Reference In"=w3196) -> ("FPGA VI Reference Out"=w3195:T31)  [unwired: 3 in, 1 out]
            n2110 = flat-sequence {
              tunnel: w3194 -> [w3199]
              tunnel: w3195 -> [w3198]
              frame #0 {
                n2111 = for "Write data to fpga memory" {
                  tunnel: w3198 -> [w3201]
                  tunnel: w3199 -> [_] mode=indexing
                  (unwired) TRUE ("Ready Write")
                  n2112 = xnode "Read/Write Control"("FPGA VI Reference In"=w3201) -> ("FPGA VI Reference Out"=w3200:T31)  [unwired: 4 in, 1 out]
                  n2113 = while {
                    tunnel: w3200 -> [w3202]
                    stop <- _ continue-if-true
                    n2114 = xnode "Read/Write Control"("FPGA VI Reference In"=w3202) -> ()  [unwired: 1 in, 3 out]
                  }
                }
                "Writing waveform to fpga memory" <- TRUE ("Writing waveform to fpga memory")
              }
              frame #1 {
                n2115 = local write "Writing waveform to fpga memory"(FALSE ("Writing waveform to fpga memory")) -> ()
              }
            }
          }
          frame Enabled {
          }
        }
        n2116 = Equal?(x=w3164, y=w3161) -> (x = y?=w3159:bool)
        n2117 = Equal?(x=w3165, y=w3161) -> (x = y?=w3160:bool)
        n2118 = Equal?(x=w3162, y=w3161) -> (x = y?=w3157:bool)
        n2119 = Equal?(x=w3163, y=w3161) -> (x = y?=w3158:bool)
        n2120 = Compound Arithmetic op=AND(w3160, w3159, w3158, w3157) -> (→"Good freq?":bool)
      }
      event "Osc trap cont.", "Osc traps", "T1 Osc Enable", "T2 Osc Enable": Value Change {
        n2121 = event-data() -> ()  [unwired: 7 out]
        n2122 = disable-structure shown="Disabled" {
          disable-tunnel: w3205 -> [w3208 _]
          frame Disabled {
            n2123 = xnode "Read/Write Control"("FPGA VI Reference In"=w3208, "Trap 1 osc enable"="T1 Osc Enable", "Trap 2 osc enable"="T2 Osc Enable") -> ()  [unwired: 1 in, 2 out]
          }
          frame Enabled {
          }
        }
      }
      event "Pressure Pump Voltage (+/-10V)": Value Change {
        n2124 = event-data() -> ()  [unwired: 7 out]
        n2125 = disable-structure shown="Disabled" {
          disable-tunnel: w3209 -> [w3213 _]
          frame Disabled {
            n2126 = Divide(x="Pressure Pump Voltage (+/-10V)", y=10.0) -> (x/y=w3210:dbl)
            n2127 = Multiply(x=w3210, y=32767.0) -> (x*y=w3211:dbl)
            n2128 = xnode "Read/Write Control"("FPGA VI Reference In"=w3213, "Pressure Pump"=w3211) -> ()  [unwired: 1 in, 2 out]
          }
          frame Enabled {
          }
        }
      }
      event "Dynamic Force FB (ronen)": Value Change {
        # "Added by ronen - for feedback on trap position by changing the actual frequency and not the set frequency - for increasing the range of feedback."
        n2129 = event-data() -> ()  [unwired: 7 out]
        n2130 = xnode "Read/Write Control"("FPGA VI Reference In"=w3217, "Dynamic Force FB (Ronen)"="Dynamic Force FB (ronen)") -> ()  [unwired: 1 in, 2 out]
      }
      event "Read Setpoint Correction File": Value Change {
        n2131 = event-data() -> ()  [unwired: 7 out]
        n2132 = local write "Read Setpoint Correction File"(FALSE ("Read Setpoint Correction File")) -> ()
        n2133 = Open/Create/Replace File(file path (use dialog)="Setpoint Correction Offset File", operation (0:open)=T40."open", access (0:read/write)=enum16{"read/write", "read-only", "write-only"}."read-only") -> (refnum out=w3241:refnum<file>)  [unwired: 1 in, 4 out]
        n2134 = Deny Access(7:w3241) -> (3:w3240:refnum<file>)  [unwired: 1 in, 2 out]
        n2135 = Read from Binary File(5:0.0, 9:T41."big-endian, network order" ("byte order (0:big-endian, network order)"), 10:-1 ("count (1)"), 11:w3240) -> (2:w3234:dbl[], 3:w3239:refnum<file>)  [unwired: 1 in, 3 out]
        n2136 = Close File(refnum=w3239) -> ()  [unwired: 1 in, 2 out]
        n2137 = Array Subset(array=w3234, index=3) -> (w3235:dbl[])  [unwired: 1 in]
        n2138 = Index Array(array=w3234, index=0) -> (element=w3223:dbl)
        n2139 = local read "T2 calibration"() -> (w3222:T5)
        n2140 = local read "T1 calibration"() -> (w3230:T6)
        n2141 = local write "Offset file step size"(w3223) -> ()
        n2142 = Unbundle By Name(w3222) -> ("T2 alpha_x (nm/V)"=w3225:dbl, "T2 kappa_x (pN/nm)"=w3224:dbl)
        n2143 = Unbundle By Name(w3230) -> ("T1 alpha_x (nm/V)"=w3227:dbl, "T1 kappa_x (pN/nm)"=w3226:dbl)
        n2144 = Multiply(x=w3227, y=w3226) -> (x*y=w3228:dbl)
        n2145 = Multiply(x=w3225, y=w3224) -> (x*y=w3229:dbl)
        n2146 = Decimate 1D Array(w3235) -> (w3232:dbl[], w3231:dbl[])  [unwired: 1 out]
        n2147 = Divide(x=w3229, y=w3228) -> (x/y=w3219:dbl)
        n2148 = property on="B factor" class="DigNum (strict)"("Val(Sgnl)"=w3219) -> ()  [unwired: 2 in, 2 out]
        n2149 = Multiply(x=w3231, y=w3219) -> (x*y=w3233:dbl[])
        n2150 = Subtract(x=w3232, y=w3233) -> (x-y=w3218:dbl[])
        n2151 = local read "Offset Values"() -> (w3221:T17)
        n2152 = Bundle By Name(cluster=w3221, "Trap 1X offset"=w3232, "Trap 2X offset"=w3231) -> (w3220:T17)
        n2153 = local write "Offset Values"(w3220) -> ()
        n2154 = property on="Setpoint offset\ncorrection values" class="Arr (strict)"("Val(Sgnl)"=w3218) -> ()  [unwired: 2 in, 2 out]
      }
      event "B factor", "Setpoint offset\ncorrection values", "Target Force (pN)": Value Change {
        w3278 = 6.0  # clock mult.
        w3279 = 49152000.0  # TCXO frequ.
        n2155 = event-data() -> ()  [unwired: 7 out]
        n2156 = local read "B factor"() -> (w3280:dbl)
        n2157 = xnode "Read/Write Control"("FPGA VI Reference In"=w3281, "B factor"=w3280) -> ("BD1 Frequency Out 1"=w3271:u64)  [unwired: 1 in, 2 out]
        n2158 = To Double Precision Float(number=w3271) -> (double precision float=w3277:dbl)
        n2159 = local read "BD 1 Frequency 2 (MHz)"() -> (w3269:dbl)
        n2160 = Multiply(x=w3279, y=w3278) -> (x*y=w3276:dbl)
        n2161 = Multiply(x=w3277, y=w3276) -> (x*y=w3275:dbl)
        n2162 = Scale By Power Of 2(n=-48, x=w3275) -> (x*2^n=w3273:dbl)
        n2163 = Divide(x=w3273, y=1000000.0) -> (x/y=w3270:dbl)
        n2164 = Subtract(x=w3269, y=w3270) -> (x-y=w3257:dbl)
        n2165 = local read "Target Force (pN)"() -> (w3268:dbl)
        n2166 = local read "T1 calibration"() -> (w3266:T6)
        n2167 = local read "Offset file step size"() -> (w3256:dbl)
        n2168 = local read "Setpoint offset\ncorrection values"() -> (w3253:dbl[])
        n2169 = Unbundle By Name(w3266) -> ("T1 alpha_x (nm/V)"=w3265:dbl, "T1 kappa_x (pN/nm)"=w3264:dbl)
        n2170 = Multiply(x=w3268, y=2.0) -> (x*y=w3262:dbl)
        n2171 = Divide(x=w3257, y=w3256) -> (x/y=w3255:dbl)
        n2172 = local read "Negate Diff?"() -> (w3259:bool)
        n2173 = To Long Integer(number=w3255) -> (32bit integer=w3254:i32)
        n2174 = Multiply(x=w3265, y=w3264) -> (x*y=w3263:dbl)
        n2175 = Index Array(array=w3253, index=w3254) -> (element=w3251:dbl)
        n2176 = Divide(x=w3262, y=w3263) -> (x/y=w3258:dbl)
        n2177 = Select(t=1, s=w3259, f=-1) -> (s? t:f=w3252:i32)
        n2178 = Multiply(x=w3252, y=w3251) -> (x*y=w3250:dbl)
        n2179 = Add(x=w3258, y=w3250) -> (x+y=w3249:dbl)
        n2180 = To Fixed-Point(number=w3249) -> (fixed-point=w3248:fxp<+/-,16,1>)  [unwired: 1 in]
        n2181 = property on="Trap Pos FB SP" class="DigNum (strict)"("Val(Sgnl)"=w3248) -> ()  [unwired: 2 in, 2 out]
      }
      event "inject shunt": Value Change {
        n2182 = event-data() -> ()  [unwired: 7 out]
        n2183 = call "hamilton_controller.vi"("Open?"="inject shunt", "valve"=enum16{"A", "B", "C", "D", "ALL"}."D", "action"=T32."MOVE VALVE") -> ("error out"=w3282:errorcluster)  [unwired: 7 in, 1 out]
      }
      event "T3 X (V)", "T3 Y (V)": Value Change {
        n2184 = event-data() -> ()  [unwired: 7 out]
        n2185 = Multiply(x="T3 X (V)", y=32767.0) -> (x*y=w3296:dbl)
        n2186 = Multiply(x="T3 Y (V)", y=32767.0) -> (x*y=w3293:dbl)
        n2187 = Divide(x=w3296, y=10.0) -> (x/y=w3297:dbl)
        n2188 = Divide(x=w3293, y=10.0) -> (x/y=w3292:dbl)
        n2189 = To Word Integer(number=w3297) -> (16bit integer=w3286:i16)
        n2190 = To Word Integer(number=w3292) -> (16bit integer=w3287:i16)
        n2191 = xnode "Read/Write Control"("FPGA VI Reference In"=w3288, "AO5"=w3286, "AO4"=w3287) -> ()  [unwired: 1 in, 2 out]
      }
    }
    "error out 2" <- w1692
    n2192 = node-c288() -> ()  [unwired: 2 out]
  }
  n2193 = node-c288() -> (w64:T35)  [unwired: 4 out]
  n2194 = timed-loop "Mouse control: trap position (AOM deflection), set confocal spot from image" {
    tunnel: [w3299] -> w69
    timing: w64 -> [_]
    timing-out: [_] -> w63
    tunnel: w21 -> [w3300]
    stop <- w3299 stop-if-true
    n2195 = node-c288() -> ()  [unwired: 2 out]
    n2196 = event shown="[0] \"Pane\": Mouse Down" {
      selector: _ -> [_ _ _ _]
      dyn-events: _ -> [_ _ _ _]
      timeout: _ -> [_ _ _ _]
      tunnel: w3300 -> [w3303 _ _ _]
      tunnel: [_ _ TRUE _] -> w3299
      event Mouse Down {
        n2197 = event-data() -> ("Time"=w3305:u32, "Coords"=w3304:T9, "Button"=w3306:u16)  [unwired: 6 out]
        n2198 = case shown="1" w3306 {
          tunnel: w3305 -> [_ _ w3412]
          tunnel: w3304 -> [_ w3343 w3410]
          tunnel: w3303 -> [_ _ w3406]
          frame 0, Default {
          }
          frame 1 {
            n2199 = property on="APD 2"() -> ("Displayed Image Size"=w3312)  [unwired: 2 in, 2 out]
            n2200 = property on="APD 1"() -> ("Displayed Image Size"=w3340)  [unwired: 2 in, 2 out]
            n2201 = property on="Detection Laser X"() -> ("Displayed Image Size"=w3341)  [unwired: 2 in, 2 out]
            n2202 = property on="Detection Laser Y"() -> ("Displayed Image Size"=w3337)  [unwired: 2 in, 2 out]
            n2203 = property on="APD 2"() -> ("Displayed Image Position"=w3313)  [unwired: 2 in, 2 out]
            n2204 = property on="APD 1"() -> ("Displayed Image Position"=w3342)  [unwired: 2 in, 2 out]
            n2205 = property on="Detection Laser X"() -> ("Displayed Image Position"=w3339)  [unwired: 2 in, 2 out]
            n2206 = property on="Detection Laser Y"() -> ("Displayed Image Position"=w3338)  [unwired: 2 in, 2 out]
            n2207 = Unbundle By Name(w3312) -> ("Width"=w3309, "Height"=w3308)
            n2208 = Unbundle By Name(w3313) -> ("Left"=w3311, "Top"=w3310)
            n2209 = Unbundle By Name(w3340) -> ("Width"=w3334, "Height"=w3333)
            n2210 = Unbundle By Name(w3341) -> ("Width"=w3330, "Height"=w3329)
            n2211 = Unbundle By Name(w3337) -> ("Width"=w3326, "Height"=w3325)
            n2212 = Unbundle By Name(w3342) -> ("Left"=w3336, "Top"=w3335)
            n2213 = Unbundle By Name(w3339) -> ("Left"=w3332, "Top"=w3331)
            n2214 = Unbundle By Name(w3338) -> ("Left"=w3328, "Top"=w3327)
            n2215 = Bundle("Left"=w3311, "Top"=w3310, "Width"=w3309, "Height"=w3308) -> (w3307:T45)  [unwired: 1 in]
            n2216 = Bundle("Left"=w3336, "Top"=w3335, "Width"=w3334, "Height"=w3333) -> (w3324:T45)  [unwired: 1 in]
            n2217 = Bundle("Left"=w3332, "Top"=w3331, "Width"=w3330, "Height"=w3329) -> (w3323:T45)  [unwired: 1 in]
            n2218 = Bundle("Left"=w3328, "Top"=w3327, "Width"=w3326, "Height"=w3325) -> (w3322:T45)  [unwired: 1 in]
